vi "Evaluate.vi"(8 "error in (no error)":errorcluster, 11 "Environment.LogFile in":refnum<class "Environment.LogFile.lvclass">) -> (0 "error out":errorcluster, 3 "Environment.LogFile out":refnum<class "Environment.LogFile.lvclass">)   [LabVIEW 2018, in "Environment.LogFile.lvclass"]
uses:
  Environment.LogFile.lvclass
  C:/Users/Colin/Documents/software_projects/labview/unit_testing_fw/Environment/Environment.lvclass
  unit_testing_fw/Environment/Environment.lvclass/Environment.ctl
  Environment.LogFile.lvclass/Environment.LogFile.ctl
  unit_testing_fw/Environment/Environment.lvclass
  <vilib>/addons/_JKI Toolkits/Caraya/classes/Assert/Assert.lvclass
  <vilib>/addons/_JKI Toolkits/Caraya/classes/Test/Test.lvclass
panel:
  # "Connector Pane"
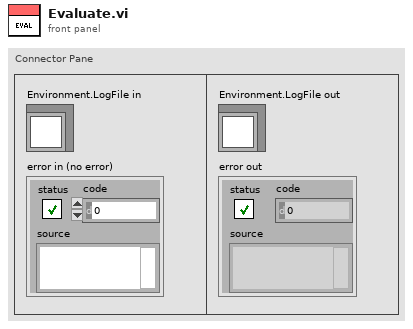
[diagram p1: front panel]
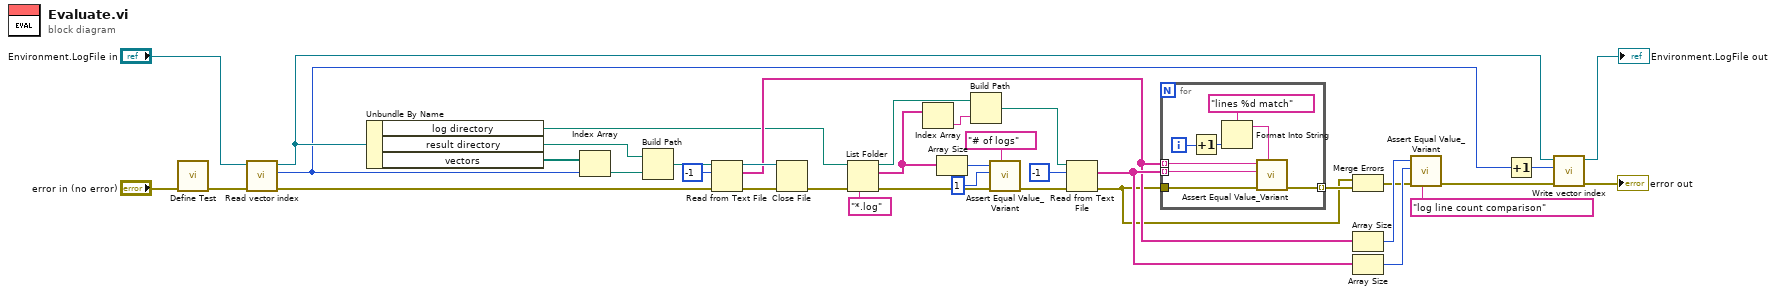
[diagram p0: block diagram]
diagram:
  n1 = call <vilib>:"Define Test.vi"("error in (no error)"="error in (no error)") -> ("error out"=w6:errorcluster)  [unwired: 9 in, 1 out]
  n2 = call "Read vector index.vi"("error in (no error)"=w6, "Environment in"="Environment.LogFile in") -> ("error out"=w29:errorcluster, "vector index"=w7:i32, "Environment out"=w36:refnum<class "Environment.LogFile.lvclass">)  [unwired: 7 in]
  n3 = Unbundle By Name(w36) -> ("log directory"=w8:path, "result directory"=w34:path, "vectors"=w35:path[])
  n4 = Index Array(array=w35, index=w7) -> (element=w33:path)
  n5 = Build Path(base path=w34, name or relative path=w33) -> (appended path=w32:path)
  n6 = Read from Text File(file (use dialog)=w32, count=-1, error in=w29) -> (refnum out=w30:refnum<file>, text=w13:string[], error out=w31:errorcluster)  [unwired: 1 in, 1 out]
  n7 = Close File(refnum=w30, error in=w31) -> (error out=w28:errorcluster)  [unwired: 1 out]
  n8 = List Folder(path=w8, pattern="*.log", error in=w28) -> (path out=w21:path, filenames=w23:string[], error out=w4:errorcluster)  [unwired: 1 in, 1 out]
  n9 = Index Array(array=w23) -> (element=w22:string)  [unwired: 1 in]
  n10 = Array Size(array=w23) -> (size(s)=w26:i32)
  n11 = Build Path(base path=w21, name or relative path=w22) -> (appended path=w20:path)
  n12 = call <vilib>:"Assert Equal Value_Variant.vi"("Label"="# of logs", "error in (no error)"=w4, "Y"=1 ("size(s)"), "X"=w26) -> ("error out"=w3:errorcluster)  [unwired: 6 in, 1 out]
  n13 = Read from Text File(file (use dialog)=w20, count=-1, error in=w3) -> (text=w14:string[], error out=w5:errorcluster)  [unwired: 1 in, 2 out]
  n14 = for {
    tunnel: w13 -> [w46] mode=indexing
    tunnel: w14 -> [w45] mode=indexing
    tunnel: w5 -> [w40]
    tunnel: [w39] -> w12 mode=indexing
    i -> [w44]
    n15 = Increment(x=w44) -> (x+1=w42:i32)
    n16 = Format Into String(format string="lines %d match" ("Label"), w42) -> (resulting string=w41:string)  [unwired: 2 in, 1 out]
    n17 = call <vilib>:"Assert Equal Value_Variant.vi"("Label"=w41, "error in (no error)"=w40, "Y"=w45, "X"=w46) -> ("error out"=w39:errorcluster)  [unwired: 6 in, 1 out]
  }
  n18 = Merge Errors(w5, w12) -> (w2:errorcluster)
  n19 = Array Size(array=w13) -> (size(s)=w17:i32)
  n20 = Array Size(array=w14) -> (size(s)=w16:i32)
  n21 = call <vilib>:"Assert Equal Value_Variant.vi"("Label"="log line count comparison", "error in (no error)"=w2, "Y"=w16, "X"=w17) -> ("error out"=w1:errorcluster)  [unwired: 6 in, 1 out]
  n22 = Increment(x=w7) -> (x+1=w10:i32)
  n23 = call "Write vector index.vi"("error in (no error)"=w1, "vector index"=w10, "Environment in"=w36) -> ("error out"=→"error out":errorcluster, "Environment out"=→"Environment.LogFile out":refnum<class "Environment.LogFile.lvclass">)  [unwired: 7 in]
